vi "Simulated VeriStand Engine.Write to HW.vi"(8 "error in (no error)":errorcluster, 11 "Simulated VeriStand Engine in":refnum<class "Simulated VeriStand Engine.lvclass">) -> (0 "error out":errorcluster, 3 "Simulated VeriStand Engine out":refnum<class "Simulated VeriStand Engine.lvclass">)   [LabVIEW 2016, in "Simulated VeriStand Engine.lvclass"]
uses:
  Simulated VeriStand Engine.lvclass
  Simulated VeriStand Engine.lvclass/Simulated VeriStand Engine.ctl
  Simulated VeriStand Custom Device/Simulated VeriStand Custom Device.lvclass
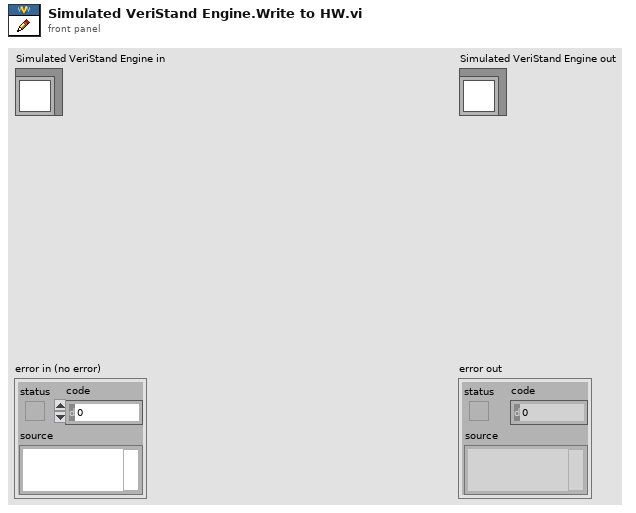
[diagram p1: front panel]
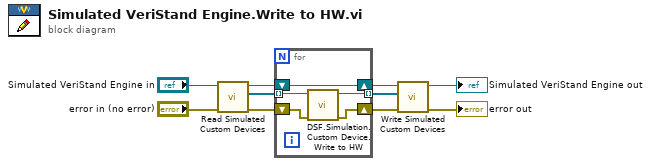
[diagram p0: block diagram]
diagram:
  n1 = call "Read Simulated Custom Devices.vi"("error in (no error)"="error in (no error)", "Simulated VeriStand Engine in"="Simulated VeriStand Engine in") -> ("error out"=w9:errorcluster, "Simulated Custom Devices"=w10:refnum<class "Simulated VeriStand Custom Device.lvclass">[], "Simulated VeriStand Engine out"=w6:refnum<class "Simulated VeriStand Engine.lvclass">)  [unwired: 7 in]
  n2 = for {
    tunnel: w10 -> [w14] mode=indexing
    shift-right: [w12] -> w7
    shift-left: w9 -> [w15]
    tunnel: [w13] -> w8 mode=indexing
    shift-right: [w11] -> w5
    shift-left: w6 -> [w11]
    n3 = call-dynamic "DSF.Simulation.Custom Device.Write to HW.vi"("error in (no error)"=w15, "Simulated VeriStand Custom Device in"=w14) -> ("error out"=w12:errorcluster, "Simulated VeriStand Custom Device out"=w13:refnum<class "Simulated VeriStand Custom Device.lvclass">)  [unwired: 8 in]
  }
  n4 = call "Write Simulated Custom Devices.vi"("error in (no error)"=w7, "Simulated Custom Devices"=w8, "Simulated VeriStand Engine in"=w5) -> ("error out"=→"error out":errorcluster, "Simulated VeriStand Engine out"=→"Simulated VeriStand Engine out":refnum<class "Simulated VeriStand Engine.lvclass">)  [unwired: 7 in]
